vi "MW_Freq_Set.vi"(8 "错误输入（无错误）":errorcluster, 10 "Set Frequency (Hz)":dbl, 11 "VISA引用句柄输入":refnum<visa-resource-name>) -> (0 "错误输出":errorcluster, 3 "VISA引用句柄输出":refnum<visa-resource-name>, 5 "Command Monitor":string)   [LabVIEW 2016, in "Microwave Source.lvlib"]
uses:
  Microwave Source.lvlib
panel:
  out "Freq (Not Verified)":dbl
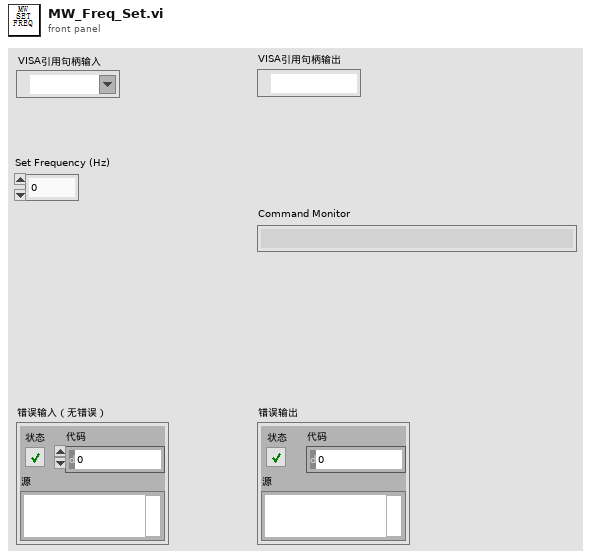
[diagram p1: front panel]
types:
  T1 = typedef "Microwave Source.lvlib/MW_ctl_DeviceType.ctl" = enum16{"R&S", "Other"}
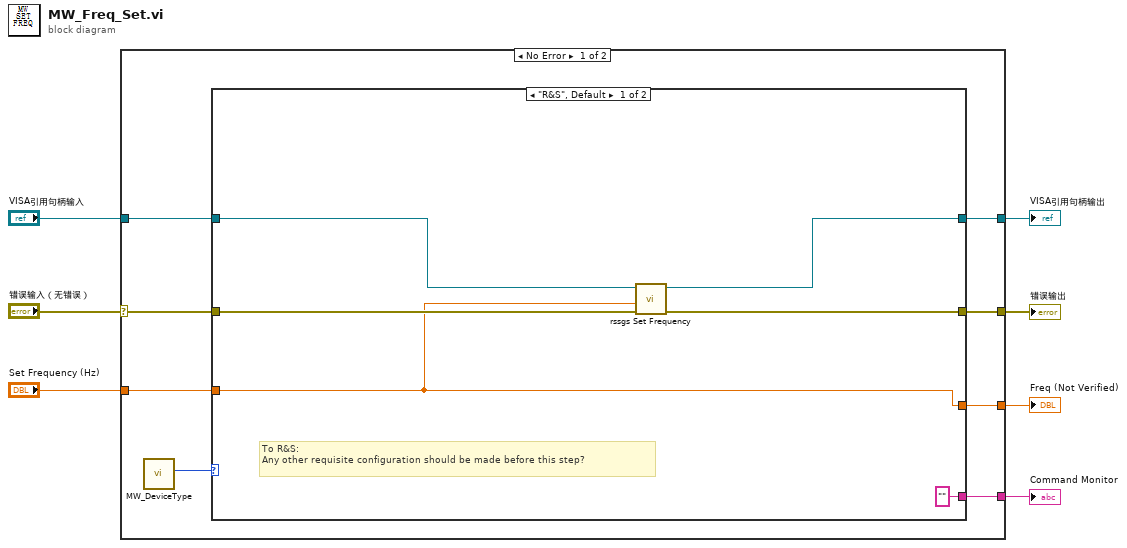
[diagram p0: block diagram]
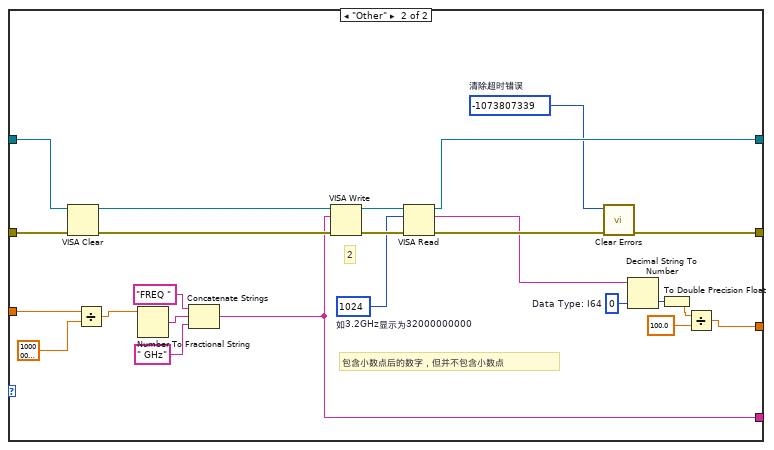
[diagram p2: hidden frame]
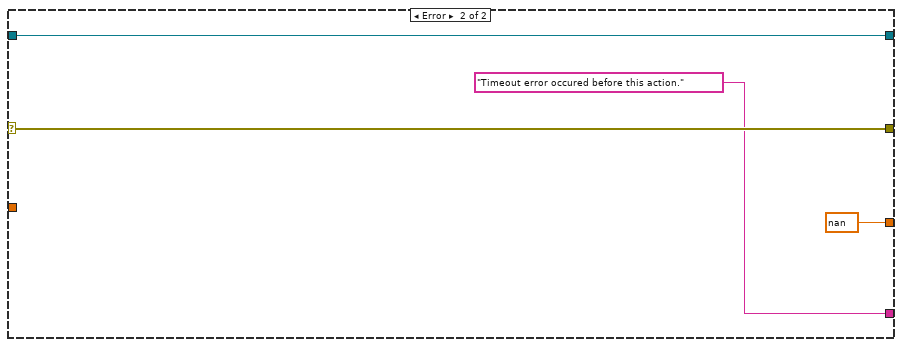
[diagram p3: hidden frame]
diagram:
  n1 = case shown="No Error" "错误输入（无错误）" {
    selector: "错误输入（无错误）" -> [w13 w49]
    tunnel: "VISA引用句柄输入" -> [w12 w48]
    tunnel: [w15 w48] -> w3
    tunnel: [w14 w49] -> w2
    tunnel: [w10 "Timeout error occured before this action." ("read buffer")] -> w4
    tunnel: [w9 nan] -> w5
    tunnel: "Set Frequency (Hz)" -> [w11 _]
    frame No Error {
      n2 = call "MW_DeviceType.vi"() -> ("DeviceType"=w8:T1)  [unwired: 11 in]
      n3 = case shown="\"R&S\", Default" w8 {
        tunnel: [w19 w44] -> w15
        tunnel: [w18 w39] -> w14
        tunnel: w13 -> [w20 w30]
        tunnel: w12 -> [w21 w29]
        tunnel: w11 -> [w17 w26]
        tunnel: ["" w25] -> w10
        tunnel: [w17 w22] -> w9
        frame "R&S", Default {
          # "To R&S:\nAny other requisite configuration should be made before this step?"
          n4 = call <instrlib>:"rssgs Set Frequency.vi"("error in (no error)"=w20, "Frequency (1.0e+6)"=w17, "VISA resource name"=w21) -> ("error out"=w18:errorcluster, "VISA resource name out"=w19:refnum<visa-resource-name>)  [unwired: 7 in]
        }
        frame "Other" {
          w37 = i64 0  # Data Type: I64
          w41 = -1073807339  # 清除超时错误
          w42 = u32 1024  # 如3.2GHz显示为32000000000
          # "包含小数点后的数字，但并不包含小数点"
          # "2"
          n5 = VISA Clear(VISA resource name=w29, error in (no error)=w30) -> (VISA resource name out=w28:refnum<visa-resource-name>, error out=w31:errorcluster)
          n6 = Divide(x=w26, y=1000000000.0 ("x")) -> (x/y=w24:dbl)
          n7 = Number To Fractional String(number=w24) -> (F-format string=w32:string)  [unwired: 3 in]
          n8 = Concatenate Strings("FREQ ", w32, " GHz") -> (w25:string)
          n9 = VISA Write(VISA resource name=w28, write buffer=w25, error in (no error)=w31) -> (VISA resource name out=w45:refnum<visa-resource-name>, error out=w43:errorcluster)  [unwired: 1 out]
          n10 = VISA Read(VISA resource name=w45, byte count=w42, error in (no error)=w43) -> (VISA resource name out=w44:refnum<visa-resource-name>, read buffer=w38:string, error out=w40:errorcluster)  [unwired: 1 out]
          n11 = call <vilib>:"Clear Errors.vi"("error in (no error)"=w40, "specific error code to clear (0: all)"=w41) -> ("error out"=w39:errorcluster)  [unwired: 4 in, 1 out]
          n12 = Decimal String To Number(string=w38, default (0L)=w37) -> (number=w36:i64)  [unwired: 1 in, 1 out]
          n13 = To Double Precision Float(number=w36) -> (double precision float=w27:dbl)
          n14 = Divide(x=w27, y=100.0) -> (x/y=w22:dbl)
        }
      }
    }
    frame Error {
    }
  }
  "Freq (Not Verified)" <- w5
  "Command Monitor" <- w4
  "错误输出" <- w2
  "VISA引用句柄输出" <- w3
